vi "DefaultSetpoints.vi"(2 "Use Defaults":bool) -> (0 "Setpoint Cluster":T1)   [LabVIEW 2011]
uses:
  2 Typedefs/setpoints to arbiter.ctl
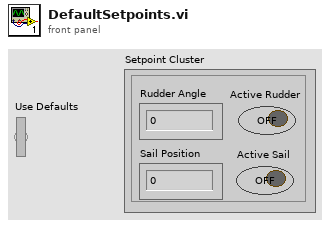
[diagram p1: front panel]
types:
  T1 = typedef "setpoints to arbiter.ctl" = cluster{"Rudder Angle":dbl, "Sail Position":dbl, "Active Rudder":bool, "Active Sail":bool}
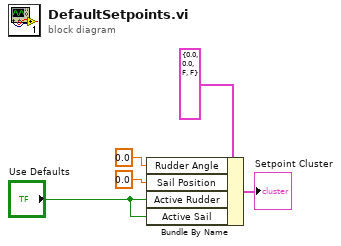
[diagram p0: block diagram]
diagram:
  n1 = Bundle By Name(cluster=T1 {"Rudder Angle"=0.0, "Sail Position"=0.0, "Active Rudder"=FALSE, "Active Sail"=FALSE} ("Setpoint Cluster"), "Rudder Angle"=0.0, "Sail Position"=0.0, "Active Rudder"="Use Defaults", "Active Sail"="Use Defaults") -> (→"Setpoint Cluster":T1)
